vi "Max Steer Voltage.vi"() -> ()   [LabVIEW 2012]
panel:
  in  "Max Steer Voltage":dbl=1.0
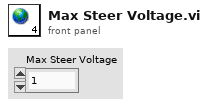
[diagram p1: front panel]
diagram:
